vi "Re-Broadcast Result.vi"(8 "error in (no error)":errorcluster, 10 "Acquired Result.lvclass":refnum<class "Acquired Result.lvclass">, 11 "Measure Object in":refnum<class "Template Module.lvclass">) -> (0 "error out":errorcluster, 3 "Measure Object out":refnum<class "Template Module.lvclass">)   [LabVIEW 2016, in "Template Module.lvclass"]
uses:
  Template Module.lvclass
  NHMFL_Core/Libraries/Instruments/Results/Acquired Result/Acquired Result.lvclass
  NHMFL_Core/Libraries/Instruments/Results/Acquired Result/Acquired Result.lvclass/Acquired Result.ctl
  Template Module Messages/Broadcast Response Msg/Broadcast Response Msg.lvclass/Broadcast Response Msg.ctl
  <vilib>/ActorFramework/Message Enqueuer/Message Enqueuer.lvclass/Message Enqueuer.ctl
  NHMFL_Core/Libraries/Instruments/Results/Acquired Result/Read Sender.vi
  <vilib>/ActorFramework/Message Enqueuer/Enqueue.vi
  Template Module Messages/Broadcast Response Msg/Broadcast Response Msg.lvclass
  C:/Program Files (x86)/National Instruments/LabVIEW 2016/vi.lib/ActorFramework/Message/Message.lvclass
  <vilib>/ActorFramework/Message Priority Queue/Priority Enqueue.vi
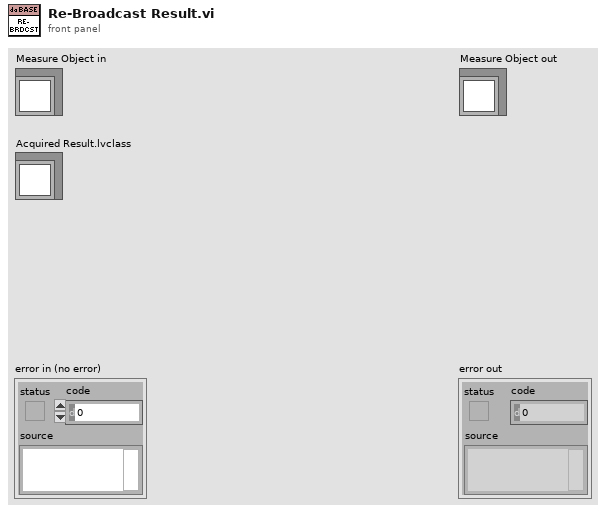
[diagram p1: front panel]
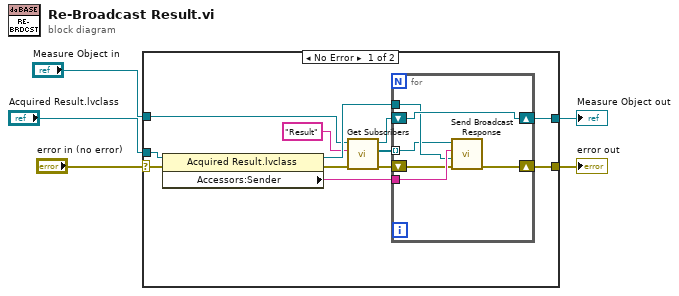
[diagram p0: block diagram]
diagram:
  n1 = case shown="No Error" "error in (no error)" {
    selector: "error in (no error)" -> [w10 w25]
    tunnel: [w9 w25] -> w4
    tunnel: [w7 w24] -> w2
    tunnel: "Measure Object in" -> [w8 w24]
    tunnel: "Acquired Result.lvclass" -> [w11 _]
    frame No Error {
      n2 = property class="Acquired Result.lvclass"(reference=w11, error in=w10) -> (reference out=w17:refnum<class "Acquired Result.lvclass">, error out=w12:errorcluster, "Accessors:Sender"=w16:string)
      n3 = call-dynamic "Get Subscribers.vi"("error in (no error)"=w12, "Topic"="Result", "Measure Object in"=w8) -> ("error out"=w15:errorcluster, "Subscribers"=w14:refnum<class "Message Enqueuer.lvclass">[], "Measure Object out"=w13:refnum<class "Template Module.lvclass">)  [unwired: 6 in]
      n4 = for {
        shift-right: [w23] -> w7
        shift-left: w13 -> [w23]
        tunnel: w14 -> [w19] mode=indexing
        shift-right: [w22] -> w9
        shift-left: w15 -> [w18]
        tunnel: w16 -> [w21]
        tunnel: w17 -> [w20]
        n5 = call "Send Broadcast Response.vi"("error in (no error)"=w18, "Acquired Result.lvclass"=w20, "Topic"=w21, "Message Enqueuer"=w19) -> ("error out"=w22:errorcluster)  [unwired: 6 in, 1 out]
      }
    }
    frame Error {
    }
  }
  "error out" <- w4
  "Measure Object out" <- w2
